vi "Test Removing Tests not In Suite.vi"(8 "error in (no error)":errorcluster, 11 "LUnit Test Suite Tests in":refnum<class "LUnit Test Suite Tests.lvclass">) -> (0 "error out":errorcluster, 3 "LUnit Test Suite Tests out":refnum<class "LUnit Test Suite Tests.lvclass">)   [LabVIEW 2020, in "LUnit Test Suite Tests.lvclass"]
uses:
  LUnit Test Suite Tests.lvclass
  C:/Program Files (x86)/National Instruments/LabVIEW 2020/vi.lib/Astemes/LUnit/Test Case.lvclass
  Test Doubles/Test Case Test Double/Test Case Test Double.lvclass
  <vilib>/Astemes/LUnit/Test Case.lvclass/Test Case.ctl
  fff43ce0-dcdd-4c3c-a466-8b369730421e.vi
  <vilib>/Astemes/LUnit/Append Pass Result.vi
  <vilib>/Astemes/LUnit/Append Fail Result.vi
  <vilib>/Astemes/LUnit/Describe Comparison.vi
  <vilib>/Astemes/LUnit/Compare Variants.vi
  <vilib>/Astemes/LUnit/Run In UI.vi
  <vilib>/Utility/error.llb/Clear Errors.vi
  source/API/LUnit Test Suite/LUnit Test Suite.lvclass
  C:/git/astemes-lunit/source/Core/Runnable/Runnable.lvclass
  <vilib>/Astemes/LUnit/Describe Variant.vi
  LUnit Test Suite Tests.lvclass/LUnit Test Suite Tests.ctl
panel:
  out "List of Runnables":string[](array[string])
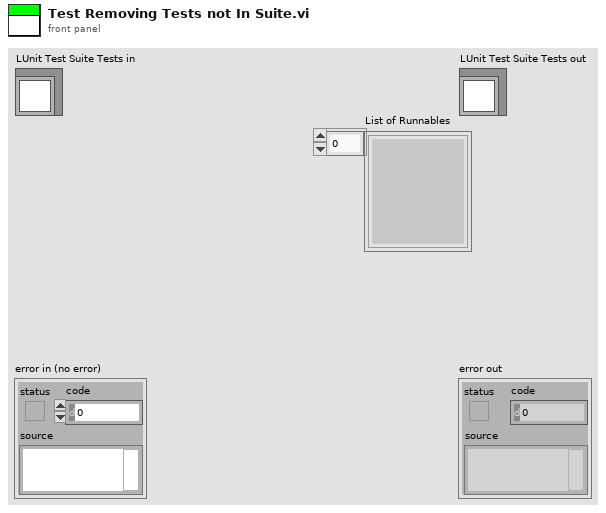
[diagram p1: front panel]
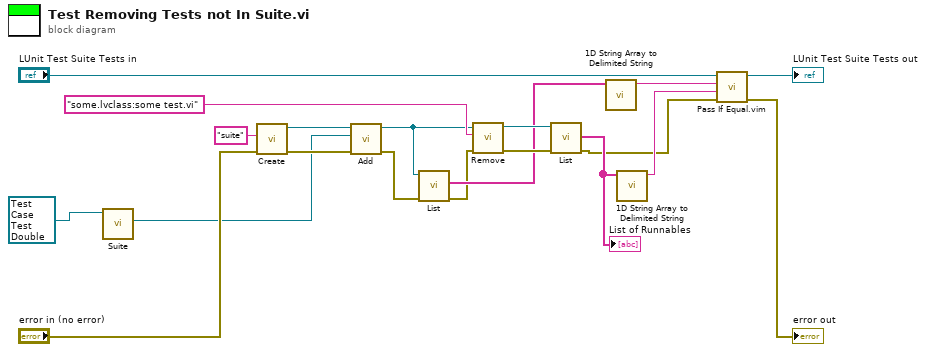
[diagram p0: block diagram]
diagram:
  n1 = call-dynamic "Suite.vi"("Test Case Class in"=refnum<class "Test Case Test Double.lvclass"> refnum ("Test Case Test Double.lvclass")) -> ("LUnit Test Suite Out"=w7:refnum<class "LUnit Test Suite.lvclass">)  [unwired: 8 in, 2 out]
  n2 = call "Create.vi"("error in (no error)"="error in (no error)", "Suite Name"="suite") -> ("error out"=w19:errorcluster, "LUnit Test Suite Out"=w6:refnum<class "LUnit Test Suite.lvclass">)  [unwired: 8 in]
  n3 = call "Add.vi"("error in (no error)"=w19, "Runnable"=w7, "LUnit Test Suite In"=w6) -> ("error out"=w2:errorcluster, "LUnit Test Suite Out"=w4:refnum<class "LUnit Test Suite.lvclass">)  [unwired: 7 in]
  n4 = call "List.vi"("error in (no error)"=w2, "LUnit Test Suite In"=w4) -> ("error out"=w1:errorcluster, "List of Runnables"=w3:string[])  [unwired: 8 in]
  n5 = call "Remove.vi"("error in (no error)"=w1, "Test to Remove"="some.lvclass:some test.vi" ("Name"), "LUnit Test Suite In"=w4) -> ("error out"=w16:errorcluster, "LUnit Test Suite Out"=w17:refnum<class "LUnit Test Suite.lvclass">)  [unwired: 7 in]
  n6 = call "List.vi"("error in (no error)"=w16, "LUnit Test Suite In"=w17) -> ("error out"=w10:errorcluster, "List of Runnables"=w12:string[])  [unwired: 8 in]
  "List of Runnables" <- w12
  n7 = call <vilib>:"1D String Array to Delimited String.vi"("string array"=w3) -> ("delimited string"=w5:string)  [unwired: 10 in]
  n8 = call <vilib>:"1D String Array to Delimited String.vi"("string array"=w12) -> ("delimited string"=w11:string)  [unwired: 10 in]
  n9 = call "Pass If Equal.vim"("error in (no error)"=w10, "Actual"=w11, "Expected"=w5, "LUnit Test Case In"="LUnit Test Suite Tests in") -> ("error out"=→"error out":errorcluster, "LUnit Test Case Out"=→"LUnit Test Suite Tests out":refnum<class "LUnit Test Suite Tests.lvclass">)  [unwired: 6 in]
